vi "权值初始.vi"() -> (2 "初始棋盘权值":sgl[][](array[numeric]))   [LabVIEW 2018]
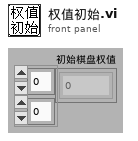
[diagram p1: front panel]
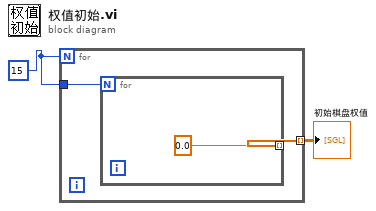
[diagram p0: block diagram]
diagram:
  w2 = 15
  n1 = for {
    N: w2 -> [_]
    tunnel: [w4] -> w1 mode=indexing
    tunnel: w2 -> [w3]
    n2 = for {
      N: w3 -> [_]
      tunnel: [sgl 0.0] -> w4 mode=indexing
    }
  }
  "初始棋盘权值" <- w1
